vi "Save_SoundFile.vi"(8 "error in":errorcluster, 10 "Binary String":string, 11 "File Path In":path) -> (0 "error out":errorcluster, 3 "File Path Out":path)   [LabVIEW 2018, in "MerriamWebsterJSON.lvlib"]
uses:
  MerriamWebsterJSON.lvlib
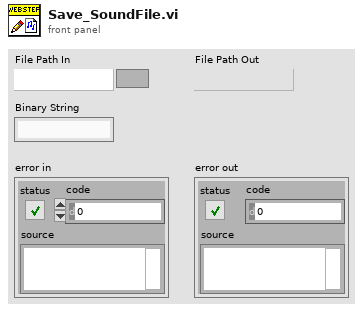
[diagram p1: front panel]
types:
  T1 = enum16{"open", "replace", "create", "open or create", "replace or create", "replace or create with confirmation"}
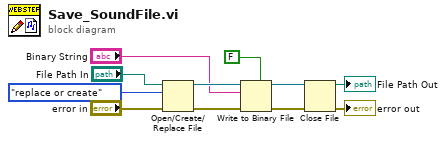
[diagram p0: block diagram]
diagram:
  n1 = Open/Create/Replace File(file path (use dialog)="File Path In", error in="error in", operation (0:open)=T1."replace or create") -> (refnum out=w11:refnum<file>, error out=w10:errorcluster)  [unwired: 3 in, 1 out]
  n2 = Write to Binary File(file (use dialog)=w11, data="Binary String", error in=w10, 5:FALSE ("prepend array or string size? (T)")) -> (refnum out=w9:refnum<file>, error out=w8:errorcluster)  [unwired: 2 in, 1 out]
  n3 = Close File(refnum=w9, error in=w8) -> (path=→"File Path Out":path, error out=→"error out":errorcluster)
